vi "ClassPanel.vi"(8 "error in (no error)":errorcluster caption="entrée d'erreur (pas d'erreur)", 11 "HeFlowMeter.lvclass":refnum<class "HeFlowMeter.lvclass">) -> (0 "error out":errorcluster caption="sortie d'erreur", 3 "HeFlowMeter.lvclass Out":refnum<class "HeFlowMeter.lvclass">)   [LabVIEW 2019, in "HeFlowMeter.lvclass"]
uses:
  HeFlowMeter.lvclass
  C:/Programmes Labview/LabscanV1A/DevicesClass/BaseDevice/BaseDevice.lvclass
  HeFlowMeter.lvclass/HeFlowMeter.ctl
  BaseDevice/ClassQueueMess.ctl
  BaseDevice/Accessor/GetClassEvent.vi
panel:
  in  "DébitMètre":u16(ring) items=["Labo Reulet", "Labo Taillefer", "Labo Pioro", "Labo Taillefer 2", "Labo Quilliam", "Labo Fournier", "Labo Dupont", "Labo Hofheinz", "Labo T.P/Juan", "Liquef. He", "Labo QFL"]
  in  "MainProgQ":refnum<queue>
  in  "MainProgQEvent":refnum<user-event>
  in  "Acq":bool
  in  "Stop":bool
  out "Débit":dbl caption="Débit m3/h" format="%.3e"
  in  "MiseAJour":bool
  out "Init Program":bool
  # "Helium FlowMeter"
  # "this MUST labeled with class name"
  # "this MUST be present and labeled \"Stop\" and \"Acq\""
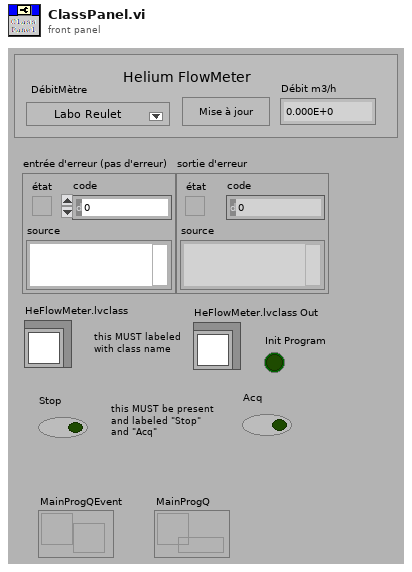
[diagram p1: front panel]
types:
  T1 = typedef "ClassQueueMess.ctl" = u16
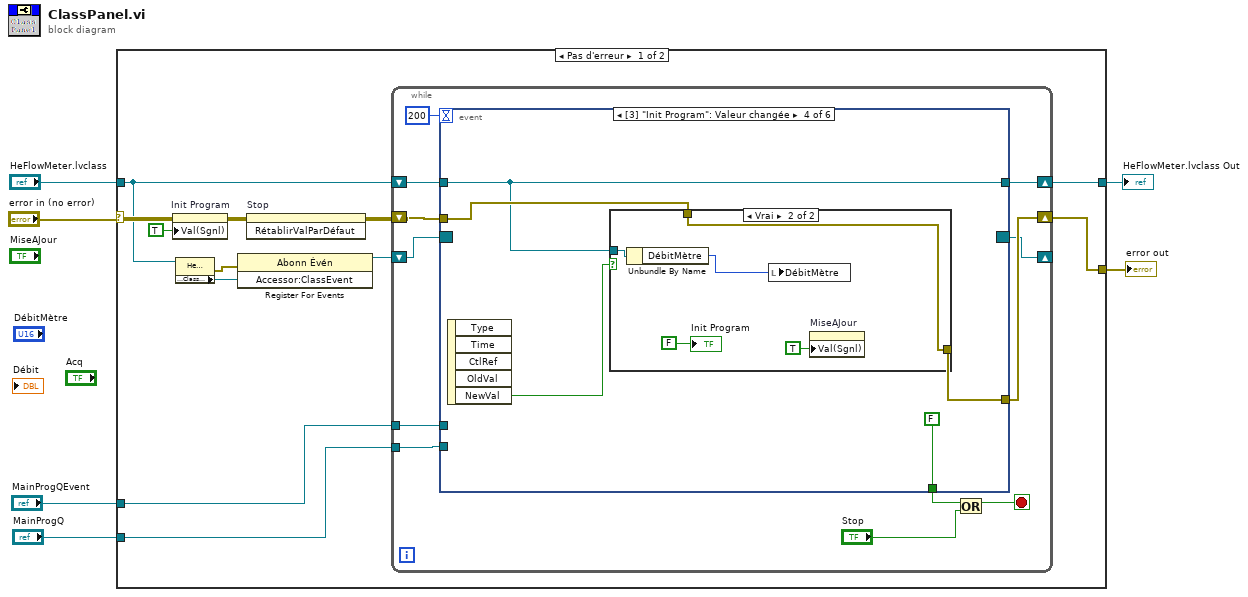
[diagram p0: block diagram]
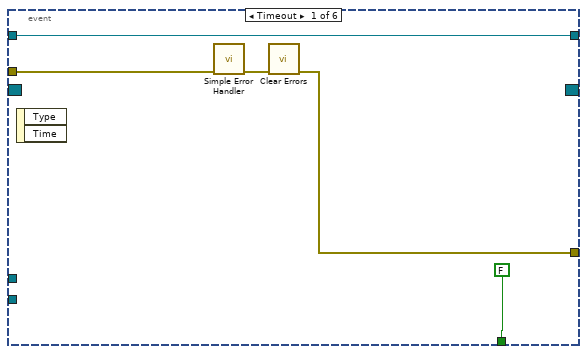
[diagram p2: hidden frame]
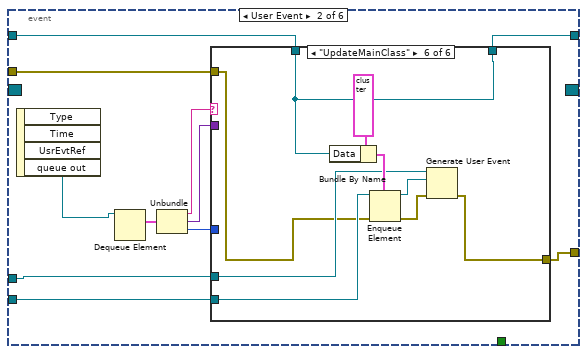
[diagram p3: hidden frame]
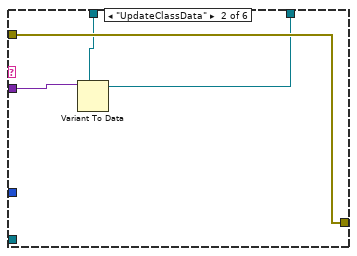
[diagram p5: hidden frame]
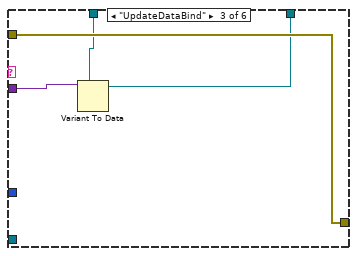
[diagram p6: hidden frame]
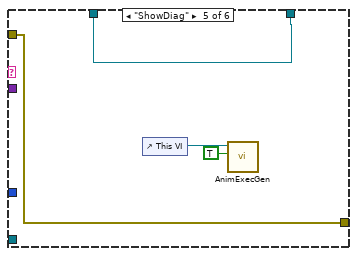
[diagram p8: hidden frame]
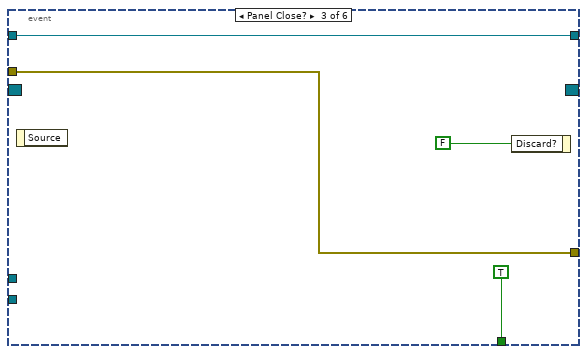
[diagram p9: hidden frame]
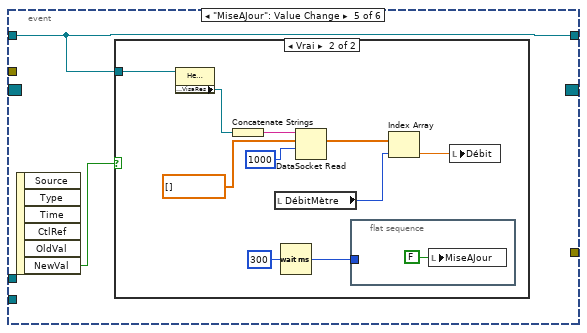
[diagram p11: hidden frame]
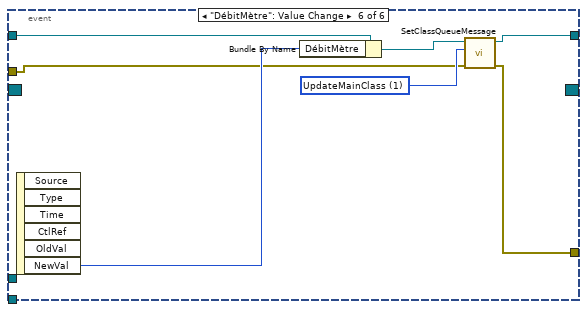
[diagram p13: hidden frame]
diagram:
  n1 = case shown="Pas d'erreur" "error in (no error)" {
    selector: "error in (no error)" -> [w15 w108]
    tunnel: [w18 w108] -> w5
    tunnel: "HeFlowMeter.lvclass" -> [w10 w107]
    tunnel: [w16 w107] -> w3
    tunnel: "MainProgQEvent" -> [w8 _]
    tunnel: "MainProgQ" -> [w7 _]
    frame No Error {
      n2 = property on="Init Program" class="Bool (strict)"(error in=w15, "Val(Sgnl)"=TRUE ("Valeur (Signalisation)")) -> (error out=w14:errorcluster)  [unwired: 1 in, 1 out]
      n3 = property class="HeFlowMeter.lvclass"(reference=w10) -> (error out=w12:errorcluster, "Accessor:ClassEvent"=w11:refnum<user-event>)  [unwired: 1 in, 1 out]
      n4 = register-events(error in=w12, w11) -> (reference out=w9:refnum<event-registration>)  [unwired: 1 in, 1 out]
      n5 = invoke on="Stop" class="Bool (strict)" method="RétablirValParDéfaut"(error in=w14) -> (error out=w13:errorcluster)  [unwired: 2 in, 2 out]
      n6 = while {
        shift-right: [w28] -> w18
        shift-left: w13 -> [w29]
        shift-right: [w25] -> w16
        shift-left: w10 -> [w27]
        shift-right: [w21] -> _
        shift-left: w9 -> [w22]
        tunnel: w8 -> [w20]
        tunnel: w7 -> [w19]
        stop <- w24 stop-if-true
        n7 = event shown="[3] \"Init Program\": Valeur changée" {
          selector: w22 -> [_ _ _ _ _ _]
          dyn-events: [_ _ _ _ _ _] -> w21
          timeout: 200 -> [_ _ _ _ _ _]
          tunnel: w29 -> [w33 w45 w73 w79 _ w101]
          tunnel: [w31 w39 w73 w78 _ w100] -> w28
          tunnel: w27 -> [w34 w46 w72 w76 w87 w106]
          tunnel: [FALSE _ TRUE FALSE _ _] -> w26
          tunnel: [w34 w38 w72 w76 w87 w103] -> w25
          tunnel: w20 -> [_ w37 _ _ _ _]
          tunnel: w19 -> [_ w36 _ _ _ _]
          event Timeout {
            n8 = event-data() -> ()  [unwired: 1 in, 2 out]
            n9 = call <vilib>:"Simple Error Handler.vi"("error in (no error)"=w33) -> ("error out"=w32:errorcluster)  [unwired: 4 in, 4 out]
            n10 = call <vilib>:"Clear Errors.vi"("error in (no error)"=w32) -> ("error out"=w31:errorcluster)  [unwired: 5 in, 1 out]
          }
          event User Event {
            n11 = event-data() -> ("queue out"=w43:refnum<queue>)  [unwired: 1 in, 3 out]
            n12 = Dequeue Element(queue=w43) -> (element=w44:cluster{"Message":string, "Data":variant, i32})  [unwired: 2 in, 3 out]
            n13 = Unbundle(w44) -> ("Message"=w42:string, "Data"=w41:variant, w40:i32)
            n14 = case shown="\"UpdateMainClass\"" w42 {
              tunnel: w45 -> [w48 w52 w56 w57 w61 w64]
              tunnel: w41 -> [_ w51 w55 _ _ _]
              tunnel: w46 -> [w47 w50 w54 w58 w62 w67]
              tunnel: [w47 w49 w53 w58 w62 w67] -> w38
              tunnel: [w48 w52 w56 w57 w61 w63] -> w39
              tunnel: w40 -> [_ _ _ _ _ _]
              tunnel: w37 -> [_ _ _ _ _ w66]
              tunnel: w36 -> [_ _ _ _ _ w65]
              frame Default {
              }
              frame "UpdateClassData" {
                n15 = Variant To Data(type=w50, Variant=w51) -> (data=w49:refnum<class "HeFlowMeter.lvclass">)  [unwired: 1 in, 1 out]
              }
              frame "UpdateDataBind" {
                n16 = Variant To Data(type=w54, Variant=w55) -> (data=w53:refnum<class "HeFlowMeter.lvclass">)  [unwired: 1 in, 1 out]
              }
              frame "MeasDone" {
              }
              frame "ShowDiag" {
                n17 = control-ref of="This VI"() -> (w60:refnum<vi>)
                n18 = call <userlib>:"AnimExecGen.vi"("Animer l'exécution ?"=TRUE, "ViRef"=w60) -> ()  [unwired: 9 in, 1 out]
              }
              frame "UpdateMainClass" {
                n19 = Bundle By Name(cluster=cluster{"Message":string, "Data":variant, i32} {"Message"="", "Data"=variant, 0} ("élément"), "Data"=w67) -> (w68:cluster{"Message":string, "Data":variant, i32})
                n20 = Enqueue Element(queue=w65, element=w68, error in (no error)=w64) -> (queue out=w71:refnum<queue>, error out=w70:errorcluster)  [unwired: 1 in, 1 out]
                n21 = Generate User Event(user event=w66, event data cluster=w71, error in=w70) -> (error out=w63:errorcluster)  [unwired: 1 in, 1 out]
              }
            }
          }
          event Panel Close? {
            n22 = event-data() -> ()  [unwired: 1 in, 1 out]
            n23 = event-data("Discard?"=FALSE ("Rejeter ?")) -> ()  [unwired: 1 in, 1 out]
          }
          event "Init Program": Value Change {
            n24 = event-data() -> ("NewVal"=w80:bool)  [unwired: 1 in, 4 out]
            n25 = case shown="Vrai" w80 {
              tunnel: w79 -> [w81 w85]
              tunnel: [w81 w85] -> w78
              tunnel: w76 -> [_ w84]
              frame False {
              }
              frame True {
                n26 = Unbundle By Name(w84) -> ("DébitMètre"=w83:u16)
                n27 = local write "DébitMètre"(w83) -> ()
                n28 = property on="MiseAJour" class="Bool (strict)"("Val(Sgnl)"=TRUE ("Valeur (Signalisation)")) -> ()  [unwired: 2 in, 2 out]
                "Init Program" <- FALSE
              }
            }
          }
          event "MiseAJour": Value Change {
            n29 = event-data() -> ("NewVal"=w88:bool)  [unwired: 1 in, 5 out]
            n30 = case shown="Vrai" w88 {
              tunnel: w87 -> [_ w95]
              frame False {
              }
              frame True {
                n31 = property class="HeFlowMeter.lvclass"(reference=w95) -> ("Accessor:VisaRes"=w94:refnum<visa-resource-name>)  [unwired: 1 in, 2 out]
                n32 = Concatenate Strings(w94) -> (w93:string)
                n33 = local read "DébitMètre"() -> (w91:u16)
                n34 = Wait (ms)(milliseconds to wait=u32 300 ("attente (ms)")) -> (millisecond timer value=w89:u32)
                n35 = DataSocket Read(9:1000 ("timeout en ms (10000)"), 10:dbl[] [], 11:w93) -> (2:w96:dbl[])  [unwired: 1 in, 7 out]
                n36 = flat-sequence {
                  tunnel: w89 -> [_]
                  frame #0 {
                    n37 = local write "MiseAJour"(FALSE ("MiseAJour")) -> ()
                  }
                }
                n38 = Index Array(array=w96, index=w91) -> (element=w92:dbl)
                n39 = local write "Débit"(w92) -> ()
              }
            }
          }
          event "DébitMètre": Value Change {
            w102 = T1 1 items=["UpdateClassData", "UpdateMainClass", "UpdateDataBind", "ReInitDevice"] ("Menu déroulant")
            n40 = event-data() -> ("NewVal"=w105:u16)  [unwired: 1 in, 5 out]
            n41 = Bundle By Name(cluster=w106, "DébitMètre"=w105) -> (w104:refnum<class "HeFlowMeter.lvclass">)
            n42 = call-dynamic "SetClassQueueMessage.vi"("ErrorIn(No Error)"=w101, "Menu déroulant"=w102, "DefaultDev.lvclass"=w104) -> ("sortie d'erreur"=w100:errorcluster, "DefaultDev.lvclass Out"=w103:refnum<class "HeFlowMeter.lvclass">)  [unwired: 7 in]
          }
        }
        n43 = Or(x=w26, y="Stop") -> (x .or. y?=w24:bool)
      }
    }
    frame Error {
    }
  }
  "error out" <- w5
  "HeFlowMeter.lvclass Out" <- w3
